vi "Queue Command Read & Parse.vi"(7 "Argument Delimiter (:)":string=":", 8 "error in":errorcluster, 9 "Q_TO":i32, 11 "Command_Q":T1) -> (0 "error out":errorcluster, 1 "Variant Data":variant, 2 "Argument":string, 3 "Command":string)   [LabVIEW 2018]
doc: "This VI waits on a Queue of type: \"Command_Queue\", which is a Command String and Variant Data. There is an option to send the commands with an argument, which is delimited with a string (default is a colon). The argument is normally used to indicate the address of the sendee, orthe object upon which to perform the command.\n\nExample: my_command:my_argument\n\nThe Timeout defaults to -1 which waits forever. If another number is wired in and the Command_Queue times out, then the returned Command string is: \"Q_Timeout\"\n(without the quotation marks)\n\nImaginatics 2006 Mike Ashe\nmichael.ashe@imaginatics.net\nCell: 860-961-0876"
uses:
  Command_Queue_Ref.ctl
  Command Queue Cluster.ctl
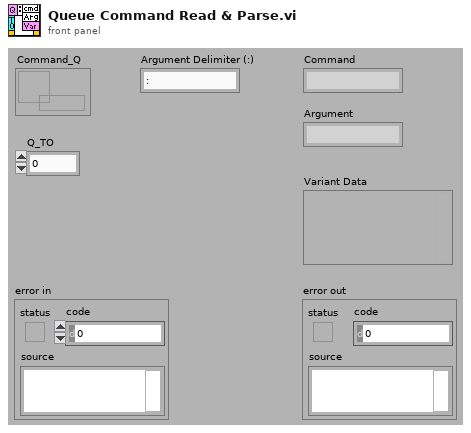
[diagram p1: front panel]
types:
  T1 = typedef "Command_Queue_Ref.ctl" = refnum<queue>
  T2 = typedef "Command Queue Cluster.ctl" = cluster{"Command":string, "Variant Data":variant}
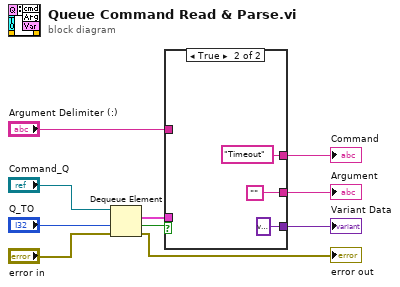
[diagram p0: block diagram]
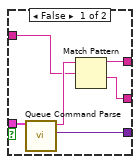
[diagram p2: hidden frame]
diagram:
  n1 = Dequeue Element(queue="Command_Q", timeout in ms (-1)="Q_TO", error in (no error)="error in") -> (element=w6:T2, timed out?=w3:bool, error out=→"error out":errorcluster)  [unwired: 1 out]
  n2 = case shown="True" w3 {
    tunnel: [w16 variant ("Variant Data")] -> w8
    tunnel: [w13 "Timeout" ("Command")] -> w7
    tunnel: w6 -> [w15 _]
    tunnel: [w12 ""] -> w2
    tunnel: "Argument Delimiter (:)" -> [w11 _]
    frame False {
      n3 = call "Queue Command Parse.vi"("command queue datatype"=w15) -> ("Variant Data"=w16:variant, "Command"=w14:string)  [unwired: 9 in]
      n4 = Match Pattern(string=w14, regular expression=w11) -> (before substring=w13:string, after substring=w12:string)  [unwired: 1 in, 2 out]
    }
    frame True {
    }
  }
  "Argument" <- w2
  "Variant Data" <- w8
  "Command" <- w7
